vi "Video_Output.vi"() -> ()   [LabVIEW 2020]
uses:
  <vilib>/Utility/miscctls.llb/LVRectTypeDef.ctl
  <vilib>/Utility/file.llb/Application Directory.vi
  <vilib>/Utility/colorconv.llb/RGB to Color.vi
  <vilib>/ptbypt/NI_PtbyPt.lvlib
panel:
  out "FPS":dbl format="%#.1f"
  out "Intensity Graph":u8[][](graph)
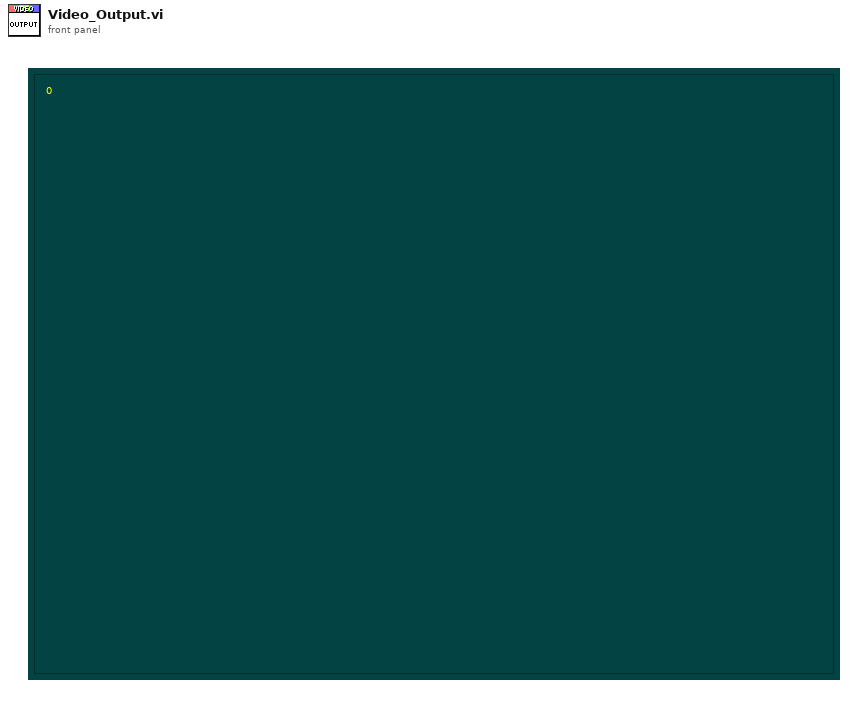
[diagram p1: front panel]
types:
  T1 = typedef "LVRectTypeDef.ctl" = cluster{"Left":i16, "Top":i16, "Right":i16, "Bottom":i16}
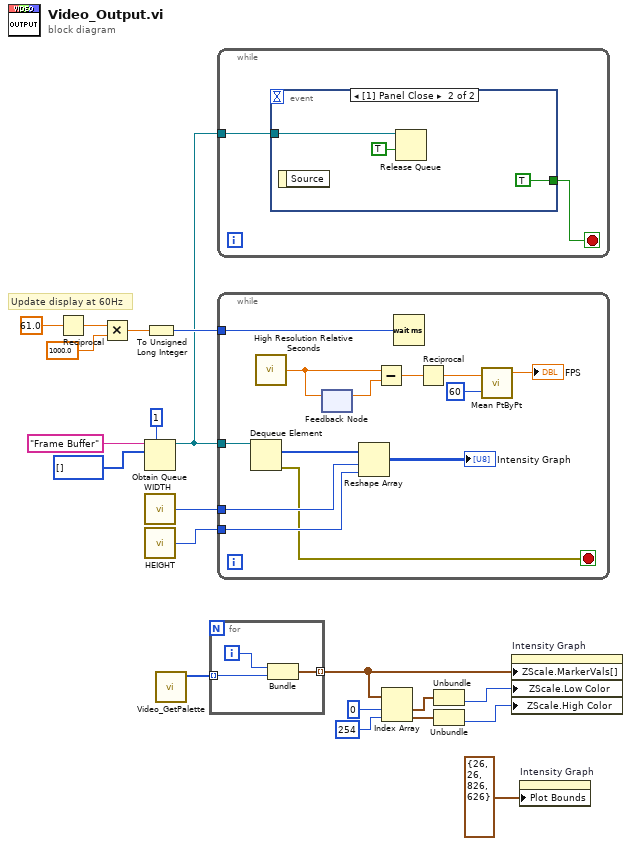
[diagram p0: block diagram]
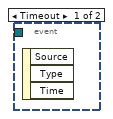
[diagram p2: hidden frame]
diagram:
  # "Update display at 60Hz"
  n1 = Reciprocal(x=61.0) -> (1/x=w16:dbl)
  n2 = Multiply(x=w16, y=1000.0) -> (x*y=w14:dbl)
  n3 = Obtain Queue(max queue size (-1, unlimited)=1, name (unnamed)="Frame Buffer", element data type=u8[] [] ("Frame Buffer")) -> (queue out=w12:refnum<queue>)  [unwired: 2 in, 2 out]
  n4 = call "WIDTH.vi"() -> ("WIDTH"=w2:i16)
  n5 = call "HEIGHT.vi"() -> ("HEIGHT"=w1:i16)
  n6 = To Unsigned Long Integer(number=w14) -> (unsigned 32bit integer=w13:u32)
  n7 = call "Video_GetPalette.vi"() -> ("Palette"=w11:u32[])  [unwired: 11 in]
  n8 = for {
    tunnel: w11 -> [w22] mode=indexing
    tunnel: [w23] -> w10 mode=indexing
    i -> [w21]
    n9 = Bundle(w21, "Color"=w22) -> (w23:cluster{i32, "Color":u32})  [unwired: 1 in]
  }
  n10 = while {
    tunnel: w12 -> [w25]
    stop <- w24 stop-if-true
    n11 = event shown="[1] Panel Close" {
      selector: _ -> [_ _]
      dyn-events: _ -> [_ _]
      timeout: _ -> [_ _]
      tunnel: w25 -> [_ w28]
      tunnel: [_ TRUE] -> w24
      event Timeout {
        n12 = event-data() -> ()  [unwired: 1 in, 3 out]
      }
      event Panel Close {
        n13 = event-data() -> ()  [unwired: 1 in, 1 out]
        n14 = Release Queue(queue=w28, force destroy? (F)=TRUE) -> ()  [unwired: 1 in, 3 out]
      }
    }
  }
  n15 = while {
    tunnel: w12 -> [w41]
    tunnel: w13 -> [w29]
    tunnel: w2 -> [w34]
    tunnel: w1 -> [w33]
    stop <- w32 stop-if-true
    n16 = Dequeue Element(queue=w41) -> (element=w30:u8[], error out=w32:errorcluster)  [unwired: 2 in, 2 out]
    n17 = call <vilib>:"High Resolution Relative Seconds.vi"() -> ("relative seconds"=w40:dbl)
    n18 = feedback-in #1(w40) -> ()
    n19 = feedback #1() -> (w39:dbl)  [unwired: 1 in]
    n20 = Reshape Array(w30, w34, w33) -> (→"Intensity Graph":u8[][])
    n21 = Subtract(x=w40, y=w39) -> (x-y=w38:dbl)
    n22 = Wait (ms)(milliseconds to wait=w29) -> ()  [unwired: 1 out]
    n23 = Reciprocal(x=w38) -> (1/x=w37:dbl)
    n24 = call <vilib>:"Mean PtByPt.vi"("x"=w37, "sample length"=60) -> ("mean"=→"FPS":dbl)  [unwired: 2 in, 1 out]
  }
  n25 = Index Array(array=w10, index #1=0 ("index"), index #2=254 ("index")) -> (element #1=w5:cluster{i32, "Color":u32}, element #2=w8:cluster{i32, "Color":u32})
  n26 = Unbundle(w5) -> ("Color"=w4:u32)  [unwired: 1 out]
  n27 = Unbundle(w8) -> ("Color"=w7:u32)  [unwired: 1 out]
  n28 = property on="Intensity Graph" class="IntGraph (strict)"("ZScale.MarkerVals[]"=w10, "ZScale.Low Color"=w4, "ZScale.High Color"=w7) -> ()  [unwired: 2 in, 2 out]
  n29 = property on="Intensity Graph" class="IntGraph (strict)"("Plot Bounds"=T1 {"Left"=26, "Top"=26, "Right"=826, "Bottom"=626} ("Plot Area Bounds")) -> ()  [unwired: 2 in, 2 out]
